vi "XML Scripter ConnPane Global.vi"() -> ()   [LabVIEW 2021]
panel:
  in  "Output Term Index":i32
  in  "Input Term Index":i32
  in  "WireThrough Bottom In Terminal":i32=7
  in  "WireThrough Bottom Out Terminal":i32=27
  in  "Available Terminals":i32[](array[numeric])=[1, 2, 3, 4, 5, 6, 8, 9, 10, 11, 12, 13]
  # "This global is used to hold available terminals and \nassociated data for the selected conn pane pattern \nin Script Source (XML).vi. For any conn pane pattern,\nwe have a preferred order for making input and \noutput connections. The array in this global represents\nthat priority order from input to output. Outputs start\nat the end of the array.\nThis global is written to in Script Source (XML).vi\nand read in Create FP Controls (XML).vi"
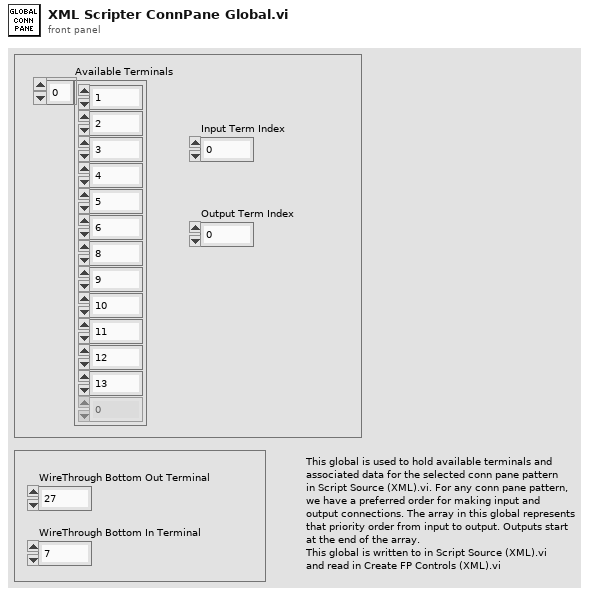
[diagram p1: front panel]
diagram:
